vi "DMM_Mixed Meas Configure and Measure.vi"(0 "DMM Handle In":refnum<k15>, 2 "Execution Option":T8, 5 "Function Settings":T6={"Range and Function"=enum."DC Voltage Auto Range", "Resolution in Digits"=5.5} {"Resolution in Digits" items=["3 1/2"=3.5, "4 1/2"=4.5, "5 1/2"=5.5, "6 1/2"=6.5, "7 1/2"=7.5]}, 7 "Timing and Trigger Settings":T3={"AC Min Frequency (Hz)"=40.0, "Aperture Time (s)"=-1.0, "Settle Time (s)"=-1.0, "Trigger Settings"={"Trigger Delay (sec)"=-1.0, "Enable Trigger?"=FALSE, "Trigger Source"=enum."Immediate", "Slope"=enum."Rising Edge"}} {"Trigger Settings"."Trigger Delay (sec)" format="%.4f"; "AC Min Frequency (Hz)" format="%.2f"}, 11 "error in":errorcluster) -> (4 "DMM Handle Out":refnum<k15>, 6 "Measurement":T1={"Measured Value"=0.0, "Out of Range"=FALSE, "Unit"="V(dc)", "Measurement"="0.0000mV (dc)"} {"Measured Value" format="%^#_9e"}, 8 "DMM Execution Settings":T2={"Absolute\nResolution"=0.0, "Input Resistance\n(Ohm)"=0.0, "Digits\nResolution"=0.0, "Range"=0.0, "Minimum\nFrequency (Hz)"=0.0, "Aperture\nTime (s)"=0.0, "Auto Range\nValue"=0.0, "Settle\nTime (s)"=0.0, "Function"=1} {"Function" items=["DC Volts"=1, "AC Volts"=2, "DC Current"=3, "AC Current"=4, "2-Wire Resistance"=5, "4-Wire Resistance"=101, "Frequency"=104, "Period"=105, "AC Volts DC Coupled"=1001, "Diode"=1002, "Waveform Voltage"=1003, "Waveform Current"=1004, "Capacitance"=1005, "Inductance"=1006, "Temperature"=108]; "Absolute\nResolution" format="%#_6p"; "Input Resistance\n(Ohm)" format="%#_6p"; "Range" format="%#_6p"; "Minimum\nFrequency (Hz)" format="%#_6p"; "Aperture\nTime (s)" format="%#_6p"; "Auto Range\nValue" format="%#_6p"; "Settle\nTime (s)" format="%#_6p"}, 15 "error out":errorcluster)   [LabVIEW 2021, in "DMM_Mixed Measurement.lvlib"]
doc: "Configures an NI-DMM measurement on the resource provided by the DMM Handle In control according to the given Function, Execution, and Timing & Trigger settings, and then executes the measurement (by default).\n\nAdditionally users can choose to Configure Only without executing the measurement or Measure Only using the existing configuration."
uses:
  DMM_Mixed Measurement.lvlib
  Common/Typedefs/Execution Options - Measure.ctl
  DMM Mixed Meas Typedefs/Function Settings.ctl
  <instrlib>/niDMM/nidmm.llb/niDMM Resolution in Digits.ctl
  DMM Mixed Meas Typedefs/Timing & Trigger Settings.ctl
  <instrlib>/niDMM/nidmm.llb/niDMM Trigger.ctl
  <instrlib>/niDMM/nidmm.llb/niDMM Slope.ctl
  DMM Mixed Meas Typedefs/DMM Execution Settings.ctl
  DMM Mixed Meas Typedefs/Measurement.ctl
  <instrlib>/niDMM/nidmm.llb/niDMM Configure Measurement Digits.vi
panel:
  # "Inputs"
  # "Outputs"
  # "Execution Settings"
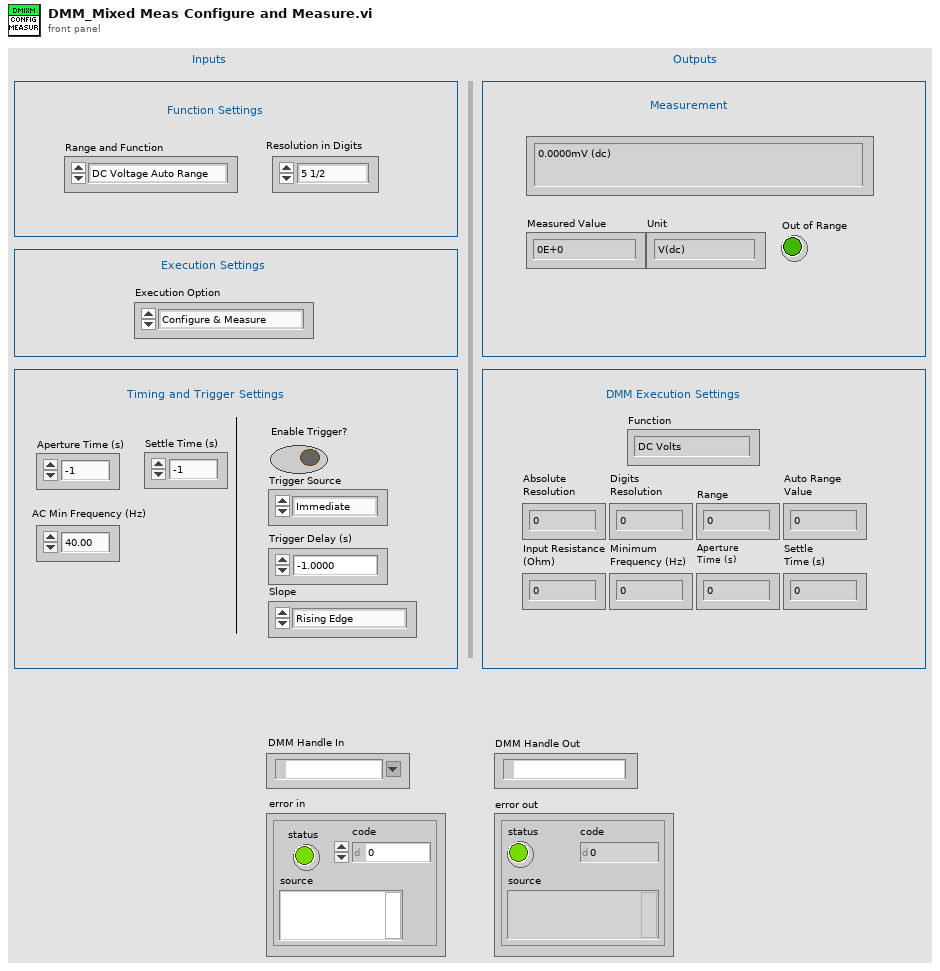
[diagram p1: front panel]
types:
  T1 = typedef "DMM_Mixed Measurement.lvlib/Measurement.ctl" = cluster{"Measured Value":dbl, "Out of Range":bool, "Unit":string, "Measurement":string}
  T2 = typedef "DMM_Mixed Measurement.lvlib/DMM Execution Settings.ctl" = cluster{"Absolute\nResolution":dbl, "Input Resistance\n(Ohm)":dbl, "Digits\nResolution":dbl, "Range":dbl, "Minimum\nFrequency (Hz)":dbl, "Aperture\nTime (s)":dbl, "Auto Range\nValue":dbl, "Settle\nTime (s)":dbl, "Function":i32}
  T3 = typedef "DMM_Mixed Measurement.lvlib/Timing & Trigger Settings.ctl" = cluster{"AC Min Frequency (Hz)":dbl, "Aperture Time (s)":dbl, "Settle Time (s)":dbl, "Trigger Settings":cluster{"Trigger Delay (sec)":dbl, "Enable Trigger?":bool, "Trigger Source":T4, "Slope":T5}}
  T4 = typedef "niDMM Trigger.ctl" = enum16{"Immediate", "External", "TTL 0", "TTL 1", "TTL 2", "TTL 3", "TTL 4", "TTL 5", "TTL 6", "Software", "TTL 7", "PXI Star", "LBR Trig 1", "Aux Trig 1"}
  T5 = typedef "niDMM Slope.ctl" = enum16{"Rising Edge", "Falling Edge"}
  T6 = typedef "DMM_Mixed Measurement.lvlib/Function Settings.ctl" = cluster{"Range and Function":enum16{"DC Voltage Auto Range", "DC 100 mV", "DC 1 V ", "DC 10 V", "DC 100 V", "DC 300 V", " ", "AC Voltage Auto Range", "AC 50 mV", "AC 200 mV", "AC 500 mV", "AC 2 V", "AC 5 V", "AC 20 V", "AC 50 V", "AC 300 V", "  ", "DC Current Auto Range", "DC 1 uA", "DC 10 uA", "DC 100 uA", "DC 1 mA", "DC 10 mA", "DC 20 mA", "DC 100 mA", "DC 200 mA", "DC 1 A", "DC 3 A", "   ", "AC Current Auto Range", "AC 100 uA", "AC 1 mA", "AC 10 mA", "AC 100 mA", "AC 500 mA", "AC 1 A", "AC 3 A", "    ", "Resistance Auto Range", "Res 100 Ohm", "Res 1 kOhm", "Res 10 kOhm", "Res 100 kOhm", "Res 1 MOhm", "Res 10 MOhm", "Res 100 MOhm", "Res 5 GOhm", "     ", "Frequency AC Auto Range", "Freq AC 50 mV", "Freq AC 500 mV", "Freq AC 5 V", "Freq AC 50 V", "Freq AC 300 V", "      ", "Period AC Auto Range", "Period AC 50 mV", "Period AC 500 mV", "Period AC 5 V", "Period AC 50 V", "Period AC 300 V"}, "Resolution in Digits":T7}
  T7 = typedef "niDMM Resolution in Digits.ctl" = dbl
  T8 = typedef "Execution Options - Measure.ctl" = enum16{"Configure & Measure", "Configure only", "Measure only"}
  T9 = typedef "niDMM Function.ctl" = enum16{"DC Volts", "AC Volts", "DC Current", "AC Current", "2-wire Resistance", "4-wire Resistance", "Diode", "Frequency", "Period", "AC Volts DC Coupled", "Capacitance", "Inductance", "Temperature"}
  T10 = cluster{"Range":dbl, "Function":T9, "AC Range":dbl, "Resolution in Digits":T7}
  T11 = cluster{"Trigger Delay (sec)":dbl, "Enable Trigger?":bool, "Trigger Source":T4, "Slope":T5}
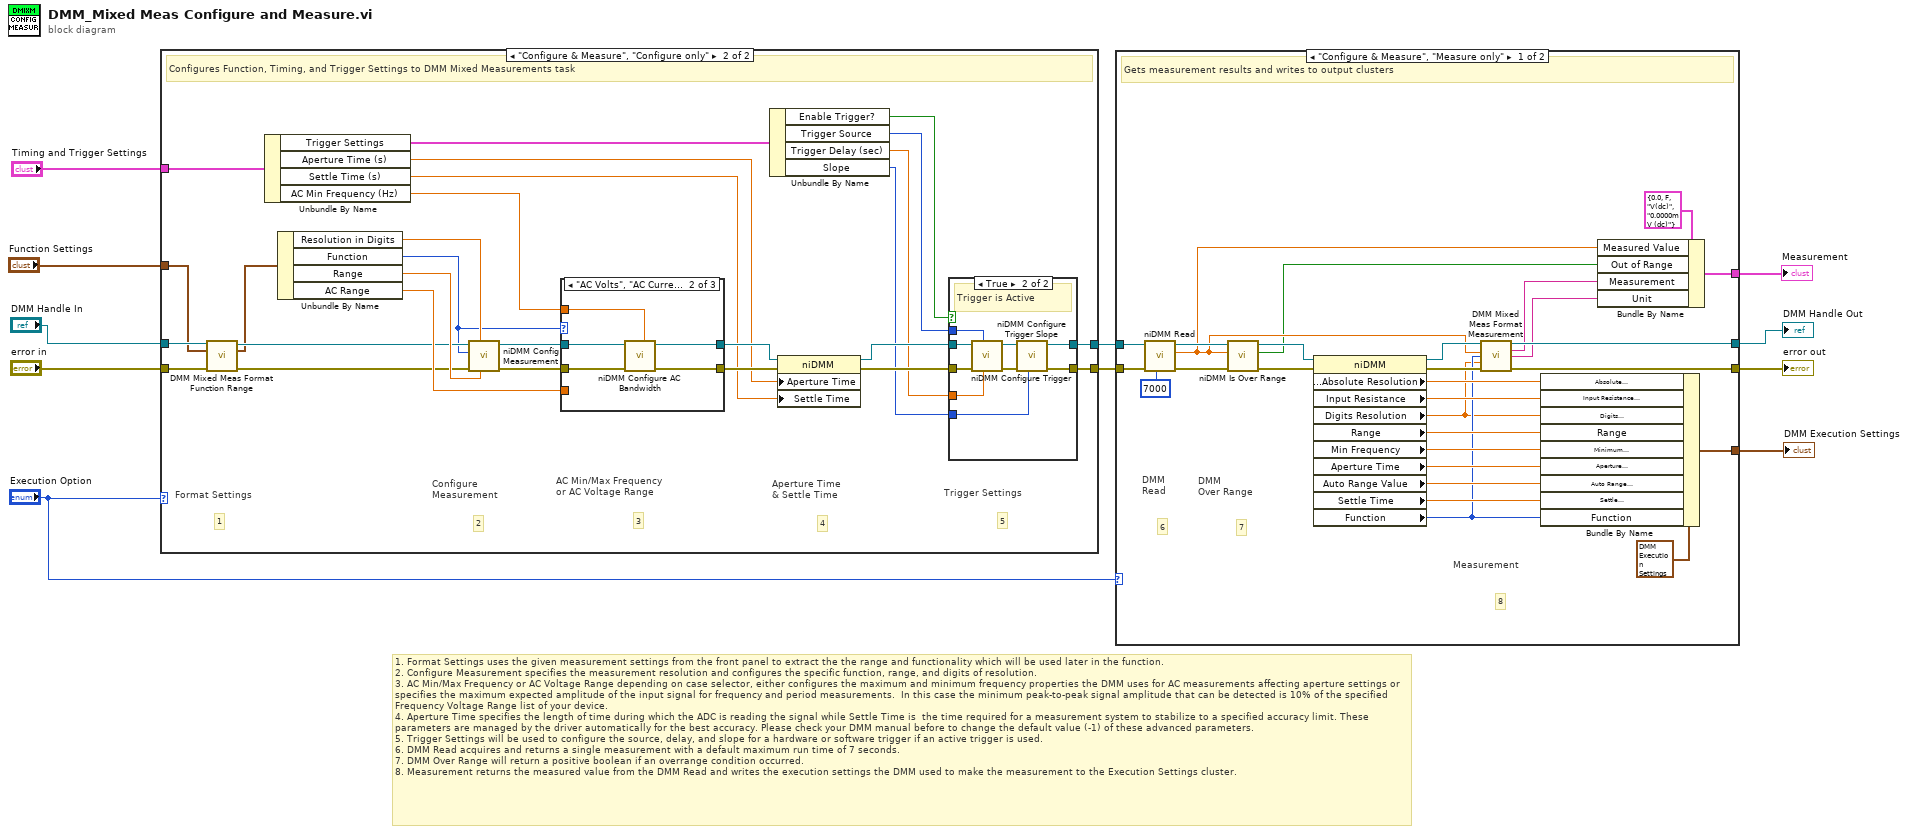
[diagram p0: block diagram]
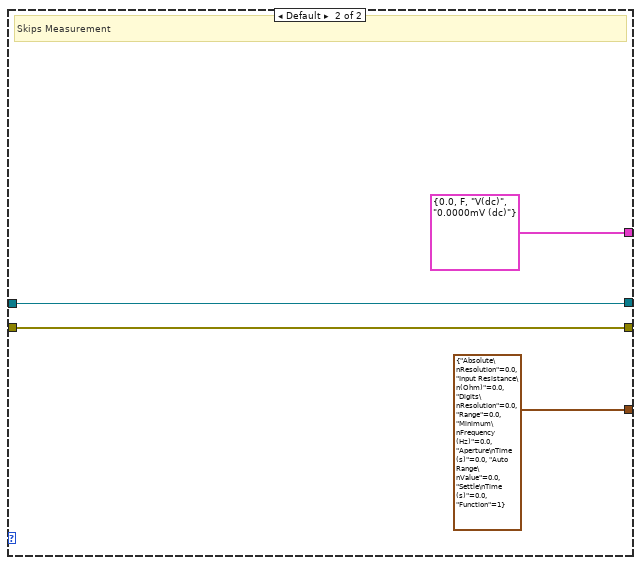
[diagram p2: hidden frame]
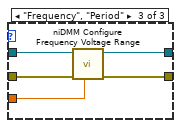
[diagram p5: hidden frame]
diagram:
  # "1. Format Settings uses the given measurement settings from the front panel to extract the the range and functionality which will be used later in the function.\n2. Configure Measurement specifies the measurement resolution and configures the specific function, range, and digits of resolution.\n3. AC Min/Max Frequency or AC Voltage Range depending on case selector, either configures the maximum and minimum frequency properties the DMM uses for AC measurements affecting aperture settings or specifies the maximum expected amplitude of the input signal for frequency and period measurements.  In this case the minimum peak-to-peak signal amplitude that can be detected is 10% of the specified Frequency Voltage Range list of your device.\n4. Aperture Time specifies the length of time during which the ADC is reading the signal while Settle Time is  the time required for a measurement system to stabilize to a specified accuracy limit. These parameters are managed by the driver automatically for the best accuracy. Please check your DMM manual before to change the default value (-1) of these advanced parameters.\n5. Trigger Settings will be used to configure the source, delay, and slope for a hardware or software trigger if an active trigger is used.\n6. DMM Read acquires and returns a single measurement with a default maximum run time of 7 seconds.\n7. DMM Over Range will return a positive boolean if an overrange condition occurred.\n8. Measurement returns the measured value from the DMM Read and writes the execution settings the DMM used to make the measurement to the Execution Settings cluster."
  n1 = case shown="\"Configure & Measure\", \"Configure only\"" "Execution Option" {
    tunnel: [w13 w38] -> w11
    tunnel: [w12 w37] -> w10
    tunnel: "Timing and Trigger Settings" -> [_ w36]
    tunnel: "DMM Handle In" -> [w13 w20]
    tunnel: "Function Settings" -> [_ w14]
    tunnel: "error in" -> [w12 w18]
    frame "Measure only" {
      # "Skips Configurations (Function, Timing and Trigger Settings)"
    }
    frame "Configure & Measure", "Configure only" {
      # "4"
      # "Aperture Time \n& Settle Time"
      # "1"
      # "Format Settings"
      # "5"
      # "3"
      # "2"
      # "Configure\nMeasurement"
      # "Trigger Settings"
      # "AC Min/Max Frequency\nor AC Voltage Range"
      # "Configures Function, Timing, and Trigger Settings to DMM Mixed Measurements task"
      n2 = call "DMM Mixed Meas Format Function Range.vi"("DMM Handle In"=w20, "Function Settings In"=w14, "error in"=w18) -> ("DMM Handle Out"=w19:refnum<k15>, "Function Settings Out"=w16:T10, "error out"=w21:errorcluster)  [unwired: 10 in]
      n3 = Unbundle By Name(w36) -> ("Trigger Settings"=w27:T11, "Aperture Time (s)"=w24:dbl, "Settle Time (s)"=w23:dbl, "AC Min Frequency (Hz)"=w22:dbl)
      n4 = Unbundle By Name(w16) -> ("Resolution in Digits"=w17:T7, "Function"=w15:T9, "Range"=w28:dbl, "AC Range"=w26:dbl)
      n5 = call-poly <instrlib>:"niDMM Config Measurement.vi"("Range"=w28, "Resolution in Digits"=w17, "error in (no error)"=w21, "Function"=w15, "instrument handle"=w19) -> ("error out"=w33:errorcluster, "instrument handle out"=w35:refnum<k15>)  [unwired: 5 in]
      n6 = case shown="\"AC Volts\", \"AC Current\"" w15 {
        tunnel: w35 -> [w42 w47 w52]
        tunnel: [w42 w46 w51] -> w34
        tunnel: w33 -> [w41 w45 w50]
        tunnel: [w41 w44 w49] -> w32
        tunnel: w22 -> [_ w43 _]
        tunnel: w26 -> [_ _ w48]
        frame Default {
        }
        frame "AC Volts", "AC Current" {
          n7 = call <instrlib>:"niDMM Configure AC Bandwidth.vi"("Min Frequency"=w43, "error in (no error)"=w45, "instrument handle"=w47) -> ("error out"=w44:errorcluster, "instrument handle out"=w46:refnum<k15>)  [unwired: 7 in]
        }
        frame "Frequency", "Period" {
          n8 = call <instrlib>:"niDMM Configure Frequency Voltage Range.vi"("Frequency Voltage Range"=w48, "error in (no error)"=w50, "instrument handle"=w52) -> ("error out"=w49:errorcluster, "instrument handle out"=w51:refnum<k15>)  [unwired: 7 in]
        }
      }
      n9 = Unbundle By Name(w27) -> ("Enable Trigger?"=w31:bool, "Trigger Source"=w30:T4, "Trigger Delay (sec)"=w29:dbl, "Slope"=w25:T5)
      n10 = property class="niDMM"(reference=w34, error in=w32, "Aperture Time"=w24, "Settle Time"=w23) -> (reference out=w39:refnum<k15>, error out=w40:errorcluster)
      n11 = case shown="True" w31 {
        tunnel: w40 -> [w53 w62]
        tunnel: w39 -> [w54 w63]
        tunnel: [w54 w57] -> w38
        tunnel: [w53 w56] -> w37
        tunnel: w30 -> [_ w60]
        tunnel: w29 -> [_ w61]
        tunnel: w25 -> [_ w55]
        frame False {
          # "No Trigger"
        }
        frame True {
          # "Trigger is Active"
          n12 = call <instrlib>:"niDMM Configure Trigger.vi"("Trigger Delay (sec)"=w61, "Trigger Source"=w60, "error in (no error)"=w62, "instrument handle"=w63) -> ("error out"=w59:errorcluster, "instrument handle out"=w58:refnum<k15>)  [unwired: 6 in]
          n13 = call <instrlib>:"niDMM Configure Trigger Slope.vi"("Slope"=w55, "error in (no error)"=w59, "instrument handle"=w58) -> ("error out"=w56:errorcluster, "instrument handle out"=w57:refnum<k15>)  [unwired: 7 in]
        }
      }
    }
  }
  n14 = case shown="\"Configure & Measure\", \"Measure only\"" "Execution Option" {
    tunnel: w11 -> [w91 w94]
    tunnel: w10 -> [w90 w95]
    tunnel: [w74 w94] -> w6
    tunnel: [w73 w95] -> w9
    tunnel: [w65 T2 {"Absolute\nResolution"=0.0, "Input Resistance\n(Ohm)"=0.0, "Digits\nResolution"=0.0, "Range"=0.0, "Minimum\nFrequency (Hz)"=0.0, "Aperture\nTime (s)"=0.0, "Auto Range\nValue"=0.0, "Settle\nTime (s)"=0.0, "Function"=1} ("Execution Settings 2")] -> w2
    tunnel: [w79 T1 {"Measured Value"=0.0, "Out of Range"=FALSE, "Unit"="V(dc)", "Measurement"="0.0000mV (dc)"}] -> w1
    frame "Configure & Measure", "Measure only" {
      # "7"
      # "DMM \nOver Range"
      # "6"
      # "DMM \nRead"
      # "8"
      # "Measurement"
      # "Gets measurement results and writes to output clusters"
      n15 = call <instrlib>:"niDMM Read.vi"("Maximum Time (msec)"=7000, "error in (no error)"=w90, "instrument handle"=w91) -> ("error out"=w88:errorcluster, "Measurement"=w68:dbl, "instrument handle out"=w89:refnum<k15>)  [unwired: 6 in]
      n16 = call <instrlib>:"niDMM Is Over Range.vi"("error in (no error)"=w88, "Measurement"=w68, "instrument handle"=w89) -> ("error out"=w86:errorcluster, "Over Range?"=w67:bool, "instrument handle out"=w87:refnum<k15>)  [unwired: 6 in]
      n17 = property class="niDMM"(reference=w87, error in=w86) -> (reference out=w76:refnum<k15>, error out=w75:errorcluster, "Configuration:Absolute Resolution"=w78:dbl, "Input Resistance"=w85:dbl, "Digits Resolution"=w69:dbl, "Range"=w84:dbl, "Min Frequency"=w83:dbl, "Aperture Time"=w82:dbl, "Auto Range Value"=w81:dbl, "Settle Time"=w80:dbl, "Function"=w70:i32)
      n18 = call "DMM Mixed Meas Format Measurement.vi"("DMM Handle In"=w76, "Measured Value"=w68, "Function"=w70, "Digits Resolution"=w69, "error in"=w75) -> ("DMM Handle Out"=w74:refnum<k15>, "Measurement"=w72:string, "Unit"=w71:string, "error out"=w73:errorcluster)  [unwired: 7 in]
      n19 = Bundle By Name(cluster=T2 {"Absolute\nResolution"=0.0, "Input Resistance\n(Ohm)"=0.0, "Digits\nResolution"=0.0, "Range"=0.0, "Minimum\nFrequency (Hz)"=0.0, "Aperture\nTime (s)"=0.0, "Auto Range\nValue"=0.0, "Settle\nTime (s)"=0.0, "Function"=1} ("Execution Settings"), "Absolute\nResolution"=w78, "Input Resistance\n(Ohm)"=w85, "Digits\nResolution"=w69, "Range"=w84, "Minimum\nFrequency (Hz)"=w83, "Aperture\nTime (s)"=w82, "Auto Range\nValue"=w81, "Settle\nTime (s)"=w80, "Function"=w70) -> (w65:T2)
      n20 = Bundle By Name(cluster=T1 {"Measured Value"=0.0, "Out of Range"=FALSE, "Unit"="V(dc)", "Measurement"="0.0000mV (dc)"}, "Measured Value"=w68, "Out of Range"=w67, "Measurement"=w72, "Unit"=w71) -> (w79:T1)
    }
    frame Default {
      # "Skips Measurement"
    }
  }
  "error out" <- w9
  "DMM Handle Out" <- w6
  "DMM Execution Settings" <- w2
  "Measurement" <- w1
